vi "表格编辑(模块版本).vi"(8 "新元素/子数组":string[](array[string]), 11 "MCListbox引用句柄":refnum<vi>) -> ()   [LabVIEW 2013]
panel:
  in  "颜色盒":u32(colorbox)=6618880
  out "表格总行数":u32=17
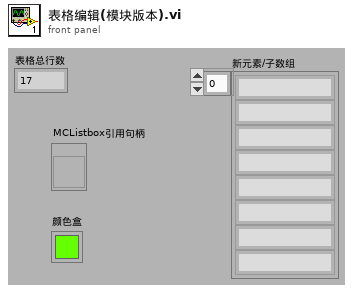
[diagram p1: front panel]
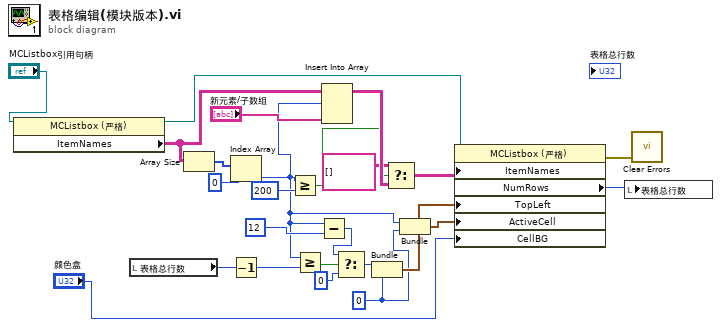
[diagram p0: block diagram]
diagram:
  w3 = 0
  n1 = property class="MCListbox (严格)"(reference="MCListbox引用句柄") -> (reference out=w22:refnum<vi>, "ItemNames"=w18:string[][])  [unwired: 1 in, 1 out]
  n2 = local read "表格总行数"() -> (w10:u32)
  n3 = Array Size(array=w18) -> (size(s)=w19:i32[])
  n4 = Index Array(array=w19, index=0 ("索引")) -> (element=w2:i32)
  n5 = Decrement(x=w10) -> (x-1=w9:u32)
  n6 = Greater Or Equal?(x=w2, y=200) -> (x >= y?=w15:bool)
  n7 = Greater Or Equal?(x=w2, y=w9) -> (x >= y?=w14:bool)
  n8 = Subtract(x=w2, y=12 ("保留行数")) -> (x-y=w11:i32)
  n9 = Insert Into Array(array=w18, index (row)=w2, new element="新元素/子数组") -> (w24:string[][])  [unwired: 1 in]
  n10 = Select(t=w11, s=w14, f=0) -> (s? t:f=w8:i32)
  n11 = Bundle("f"=w8, w3) -> (w5:cluster{"f":i32, i32})  [unwired: 1 out]
  n12 = Select(t=string[][] [], s=w15, f=w24) -> (s? t:f=w21:string[][])
  n13 = Bundle(w2, w3) -> (w4:cluster{i32, i32})  [unwired: 1 out]
  n14 = property class="MCListbox (严格)"(reference=w22, "ItemNames"=w21, "TopLeft"=w5, "ActiveCell"=w4, "CellBG"="颜色盒") -> (error out=w6:errorcluster, "NumRows"=w7:u32)  [unwired: 1 in, 1 out]
  n15 = local write "表格总行数"(w7) -> ()
  n16 = call <vilib>:"Clear Errors.vi"("error in (no error)"=w6) -> ()  [unwired: 7 out]
